vi "AB_RW_Project_Build_Info.vi"(7 "action":T1, 8 "error in (no error)":errorcluster, 10 "buildInfo in":T2, 11 "Object In":T3) -> (0 "error out":errorcluster, 2 "buildInfo out":T2, 3 "Object Out":T3)   [LabVIEW 2020]
uses:
  <resource>/Framework/Providers/API/ItemRef.ctl
  <vilib>/AppBuilder/RW_Project/AB_RW_Project_Build_Data.ctl
  <vilib>/AppBuilder/RW_Project/AB_RW_Project_PropBag_Action.ctl
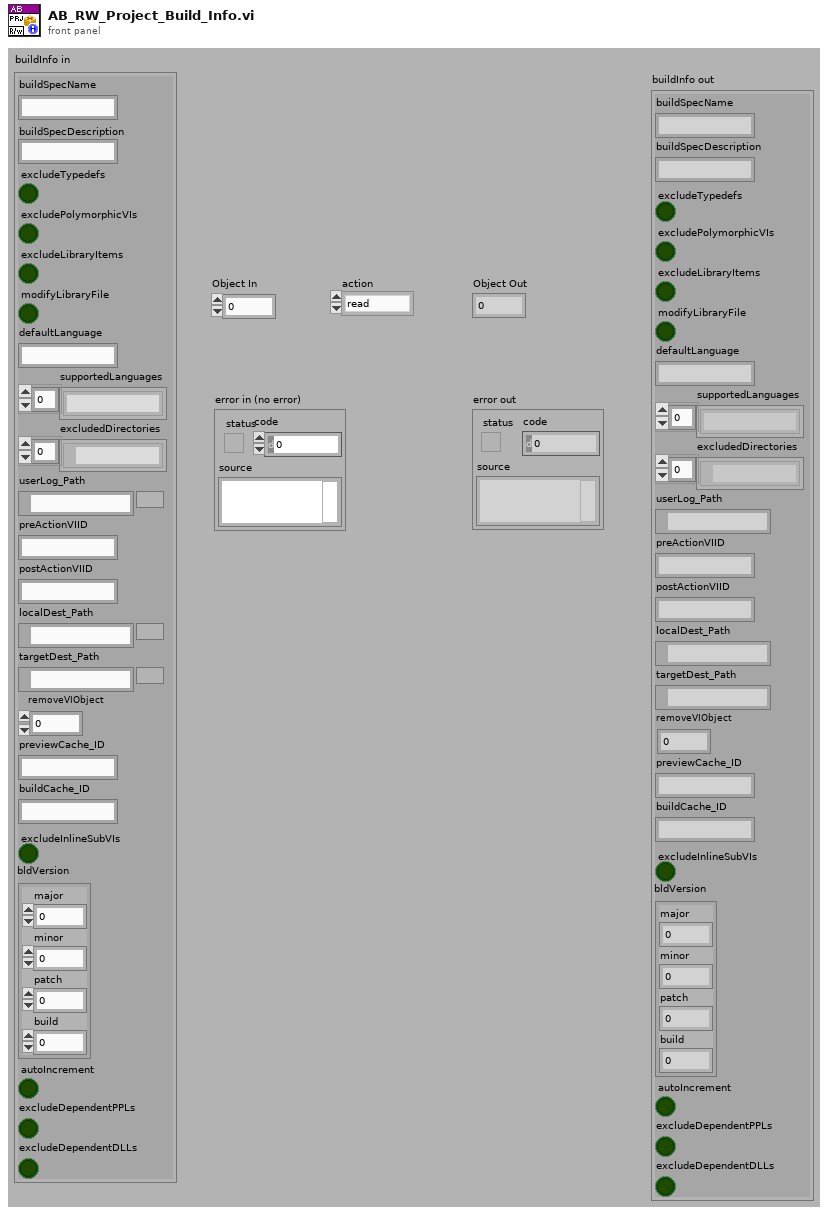
[diagram p1: front panel]
types:
  T1 = typedef "AB_RW_Project_PropBag_Action.ctl" = enum16{"read", "write", "clear", "readPrevious", "writePrevious", "clearPrevious"}
  T2 = typedef "AB_RW_Project_Build_Data.ctl" = cluster{"buildSpecName":string, "buildSpecDescription":string, "excludeTypedefs":bool, "excludePolymorphicVIs":bool, "excludeLibraryItems":bool, "modifyLibraryFile":bool, "defaultLanguage":string, "supportedLanguages":string[], "excludedDirectories":path[], "userLog_Path":path, "preActionVIID":string, "postActionVIID":string, "localDest_Path":path, "targetDest_Path":path, "removeVIObject":u16, "previewCache_ID":string, "buildCache_ID":string, "excludeInlineSubVIs":bool, "bldVersion":cluster{"major":u16, "minor":u16, "patch":u16, "build":u16}, "autoIncrement":bool, "excludeDependentPPLs":bool, "excludeDependentDLLs":bool}
  T3 = typedef "ItemRef.ctl" = u64
  T4 = cluster{"[0]":i32, "[1]":i32, "[2]":i32, "[3]":i32}
  T5 = cluster{"major":u16, "minor":u16, "patch":u16, "build":u16}
  T6 = typedef "AB_Relative_Path_Type.ctl" = enum16{"<none>", "relativeToCommon", "relativeToAppDir", "relativeToProject"}
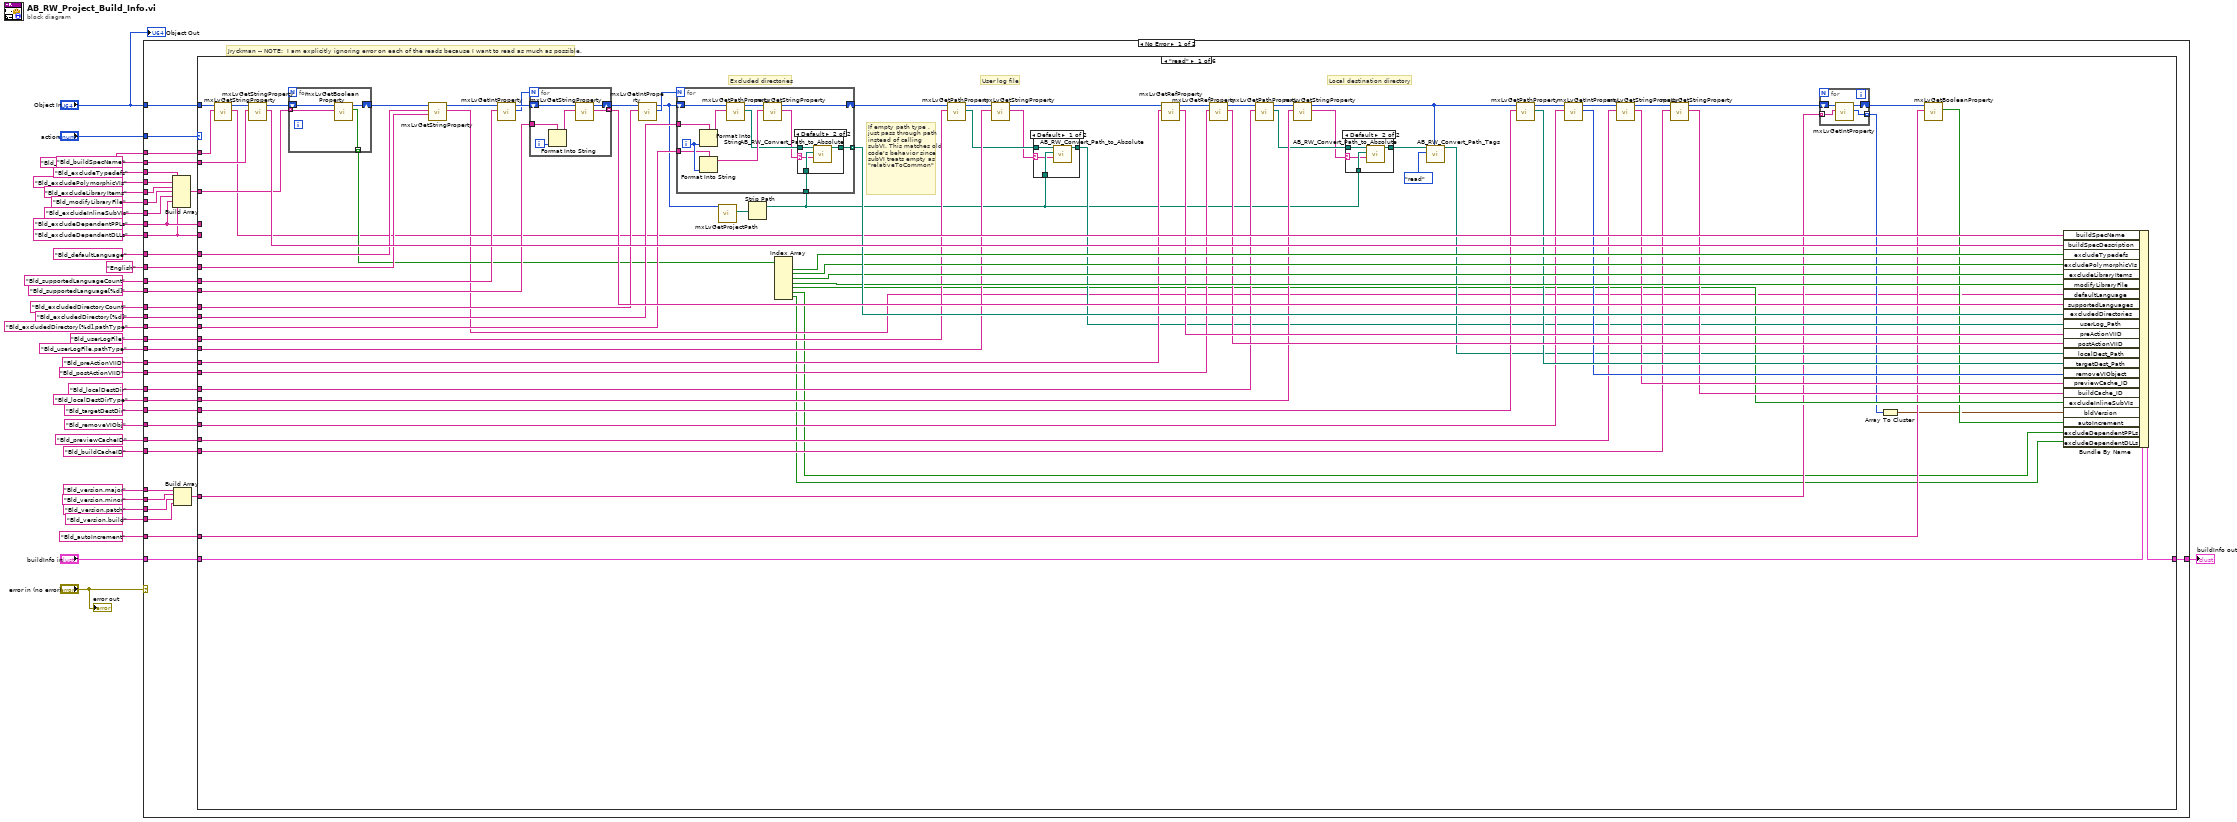
[diagram p0: block diagram]
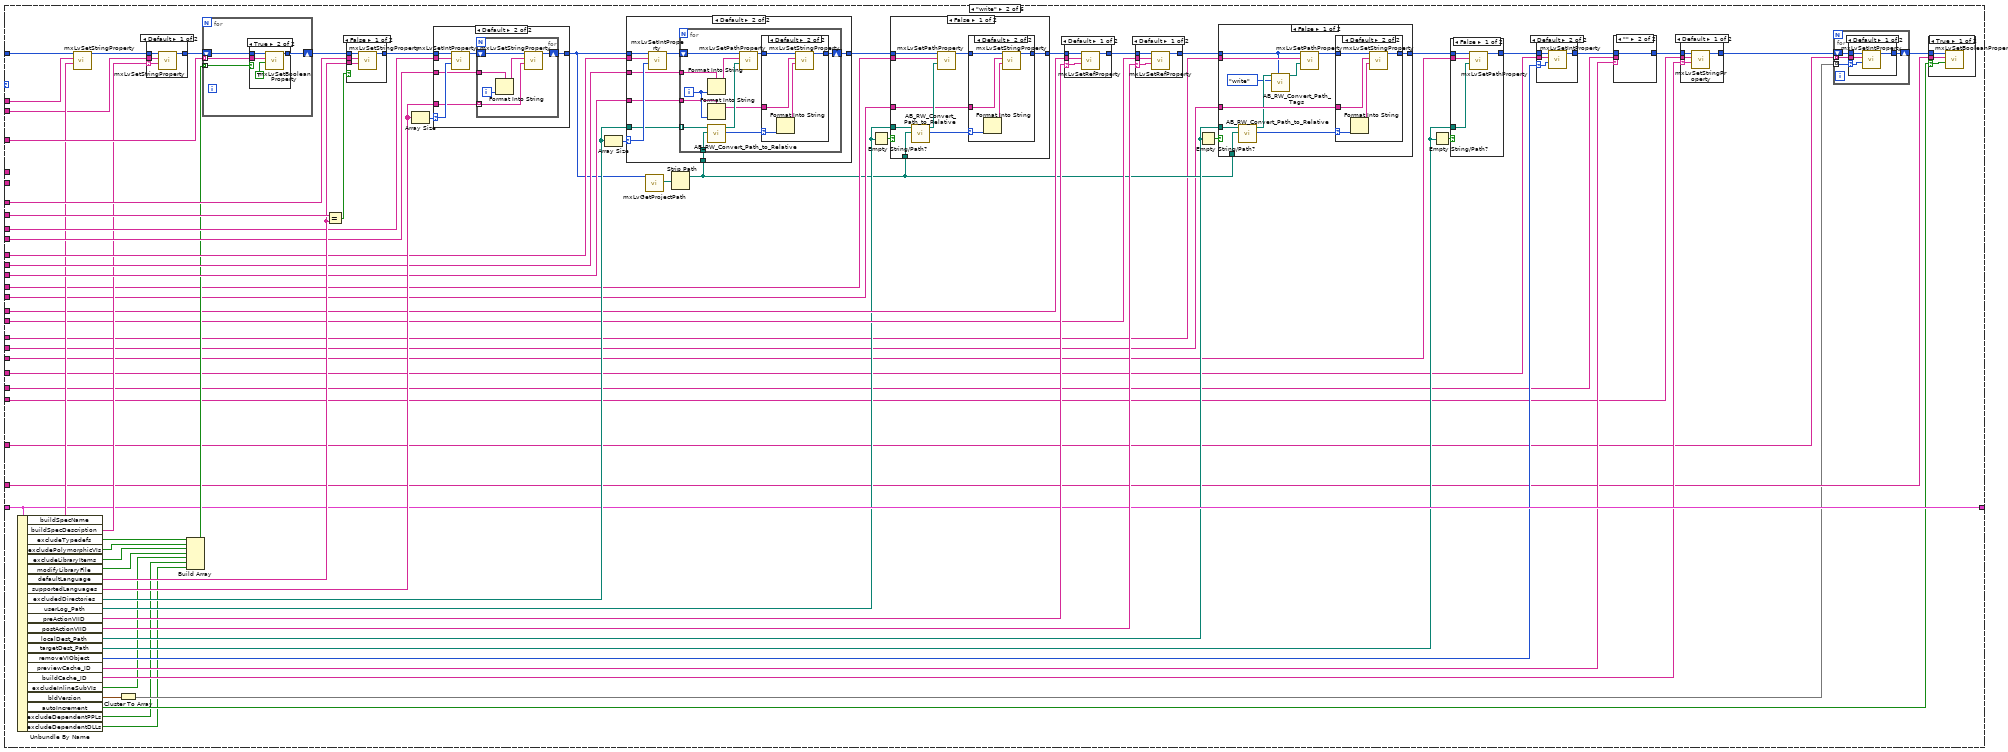
[diagram p5: hidden frame]
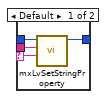
[diagram p9: hidden frame]
diagram:
  n1 = case shown="No Error" "error in (no error)" {
    tunnel: "Object In" -> [w73 _]
    tunnel: [w62 _] -> w34
    tunnel: "Bld_buildSpecDescription" ("Tag") -> [w72 _]
    tunnel: "Bld_excludeTypedefs" ("Tag") -> [w58 _]
    tunnel: "Bld_defaultLanguage" ("Tag") -> [w71 _]
    tunnel: "English" ("Tag") -> [w70 _]
    tunnel: "Bld_supportedLanguageCount" ("Tag") -> [w69 _]
    tunnel: "Bld_supportedLanguage[%d]" ("Tag") -> [w68 _]
    tunnel: "Bld_excludedDirectoryCount" ("Tag") -> [w67 _]
    tunnel: "Bld_excludedDirectory[%d]" ("Tag") -> [w66 _]
    tunnel: "Bld_excludedDirectory[%d].pathType" ("Tag") -> [w65 _]
    tunnel: "buildInfo in" -> [w64 _]
    tunnel: "action" -> [w63 _]
    tunnel: "Bld_excludePolymorphicVIs" ("Tag") -> [w61 _]
    tunnel: "Bld_excludeLibraryItems" ("Tag") -> [w60 _]
    tunnel: "Bld_modifyLibraryFile" ("Tag") -> [w59 _]
    tunnel: "Bld_buildSpecName" ("Tag") -> [w56 _]
    tunnel: "Bld_userLogFile" ("Tag") -> [w55 _]
    tunnel: "Bld_userLogFile.pathType" ("Tag") -> [w54 _]
    tunnel: "Bld_preActionVIID" ("Tag") -> [w53 _]
    tunnel: "Bld_postActionVIID" ("Tag") -> [w52 _]
    tunnel: "Bld_localDestDir" ("Tag") -> [w51 _]
    tunnel: "Bld_targetDestDir" ("Tag") -> [w50 _]
    tunnel: "Bld_localDestDirType" ("Tag") -> [w49 _]
    tunnel: "Bld_removeVIObj" ("Tag") -> [w48 _]
    tunnel: "Bld_previewCacheID" ("Tag") -> [w47 _]
    tunnel: "Bld_buildCacheID" ("Tag") -> [w46 _]
    tunnel: "Bld_excludeInlineSubVIs" ("Tag") -> [w45 _]
    tunnel: "Bld_version.major" ("Tag") -> [w43 _]
    tunnel: "Bld_version.minor" ("Tag") -> [w42 _]
    tunnel: "Bld_version.patch" ("Tag") -> [w40 _]
    tunnel: "Bld_version.build" ("Tag") -> [w41 _]
    tunnel: "Bld_autoIncrement" ("Tag") -> [w44 _]
    tunnel: "Bld_excludeDependentPPLs" ("Tag") -> [w38 _]
    tunnel: "Bld_excludeDependentDLLs" ("Tag") -> [w37 _]
    frame No Error {
      # "Jryckman -- NOTE:  I am explicitly ignoring error on each of the reads because I want to read as much as possible."
      n2 = Build Array(w58, w61, w60, w59, w45, w38, w37) -> (w57:string[])
      n3 = Build Array(w43, w42, w40, w41) -> (w39:string[])
      n4 = case shown="\"read\"" w63 {
        tunnel: w73 -> [w125 w242 w440 w465 w470 w483]
        tunnel: w72 -> [w151 w237 w442 _ _ _]
        tunnel: w71 -> [w149 w262 w441 _ _ _]
        tunnel: w70 -> [w148 w261 _ _ _ _]
        tunnel: w69 -> [w146 w256 w439 _ _ _]
        tunnel: w68 -> [w143 w255 w436 _ _ _]
        tunnel: w67 -> [w140 w251 w432 _ _ _]
        tunnel: w66 -> [w138 w250 w431 _ _ _]
        tunnel: w65 -> [w137 w249 w430 _ _ _]
        tunnel: w64 -> [w134 w221 w427 w467 w471 w484]
        tunnel: [w135 w221 w427 w466 w471 w484] -> w62
        tunnel: w57 -> [w131 w243 w426 _ _ _]
        tunnel: w56 -> [w123 w240 w425 _ _ _]
        tunnel: w55 -> [w118 w234 w423 _ _ _]
        tunnel: w54 -> [w116 w230 w421 _ _ _]
        tunnel: w53 -> [w115 w228 w418 _ _ _]
        tunnel: w52 -> [w112 w225 w417 _ _ _]
        tunnel: w51 -> [w107 w216 w414 _ _ _]
        tunnel: w50 -> [w105 w214 w412 _ _ _]
        tunnel: w49 -> [w106 w217 w413 _ _ _]
        tunnel: w48 -> [w101 w210 w409 w464 w469 w482]
        tunnel: w47 -> [w99 w207 w407 _ _ _]
        tunnel: w46 -> [w96 w204 w405 _ _ _]
        tunnel: w44 -> [w79 w198 w401 _ _ _]
        tunnel: w39 -> [w81 w195 w403 _ _ _]
        tunnel: w38 -> [_ _ _ _ _ w479]
        tunnel: w37 -> [_ _ _ _ _ w478]
        frame "read" {
          # "If empty path type , just pass through path instead of calling subVI. This matches old code's behavior since subVI treats empty as \"relativeToCommon\""
          # "Local destination directory"
          # "User log file"
          # "Excluded directories"
          n5 = call <resource>:"mxLvGetStringProperty.vi"("Tag"=w123, "Item"=w125) -> ("Value"=w122:string, "Item"=w124:T3)  [unwired: 1 in, 7 out]
          n6 = call <resource>:"mxLvGetStringProperty.vi"("Tag"=w151, "Item"=w124) -> ("Value"=w150:string, "Item"=w133:T3)  [unwired: 1 in, 7 out]
          n7 = for {
            shift-right: [w169] -> w132
            shift-left: w133 -> [w167]
            tunnel: w131 -> [w168] mode=indexing
            tunnel: [w166] -> w130 mode=indexing
            n8 = call <resource>:"mxLvGetBooleanProperty.vi"("Tag"=w168, "Item"=w167) -> ("Value"=w166:bool, "Item"=w169:T3)  [unwired: 1 in, 7 out]
          }
          n9 = call <resource>:"mxLvGetStringProperty.vi"("Default Value (\"\")"=w148, "Tag"=w149, "Item"=w132) -> ("Value"=w76:string, "Item"=w147:T3)  [unwired: 1 in, 6 out]
          n10 = call <resource>:"mxLvGetIntProperty.vi"("Tag"=w146, "Item"=w147) -> ("Value"=w144:i32, "Item"=w145:T3)  [unwired: 1 in, 7 out]
          n11 = for {
            N: w144 -> [_]
            shift-right: [w189] -> w141
            shift-left: w145 -> [w190]
            tunnel: w143 -> [w191]
            tunnel: [w187] -> w142 mode=indexing
            i -> [w192]
            n12 = Format Into String(format string=w191, w192) -> (resulting string=w188:string)  [unwired: 2 in, 1 out]
            n13 = call <resource>:"mxLvGetStringProperty.vi"("Tag"=w188, "Item"=w190) -> ("Value"=w187:string, "Item"=w189:T3)  [unwired: 1 in, 7 out]
          }
          n14 = call <resource>:"mxLvGetIntProperty.vi"("Tag"=w140, "Item"=w141) -> ("Value"=w139:i32, "Item"=w121:T3)  [unwired: 1 in, 7 out]
          n15 = call <resource>:"mxLvGetProjectPath.vi"("Item"=w121) -> ("Project Path"=w120:path)  [unwired: 1 in, 9 out]
          n16 = Strip Path(path=w120) -> (stripped path=w86:path)  [unwired: 1 out]
          n17 = for {
            N: w139 -> [_]
            shift-right: [w174] -> w119
            shift-left: w121 -> [w178]
            tunnel: w138 -> [w181]
            tunnel: w137 -> [w179]
            tunnel: w86 -> [w171]
            tunnel: [w172] -> w136 mode=indexing
            i -> [w180]
            n18 = Format Into String(format string=w181, w180) -> (resulting string=w177:string)  [unwired: 2 in, 1 out]
            n19 = Format Into String(format string=w179, w180) -> (resulting string=w175:string)  [unwired: 2 in, 1 out]
            n20 = call <resource>:"mxLvGetPathProperty.vi"("Tag"=w177, "Item"=w178) -> ("Path"=w173:path, "Item"=w176:T3)  [unwired: 2 in, 6 out]
            n21 = call <resource>:"mxLvGetStringProperty.vi"("Tag"=w175, "Item"=w176) -> ("Value"=w170:string, "Item"=w174:T3)  [unwired: 1 in, 7 out]
            n22 = case shown="Default" w170 {
              selector: w170 -> [_ w183]
              tunnel: w173 -> [w182 w186]
              tunnel: [w182 w185] -> w172
              tunnel: w171 -> [_ w184]
              frame "" {
              }
              frame Default {
                n23 = call <vilib>:"AB_RW_Convert_Path_to_Absolute.vi"("relativeType"=w183, "commonPath"=w184, "relativePath"=w186) -> ("absolute path"=w185:path)  [unwired: 7 in, 1 out]
              }
            }
          }
          n24 = Index Array(array=w130) -> (element #1=w129:bool, element #2=w128:bool, element #3=w127:bool, element #4=w126:bool, element #5=w83:bool, element #6=w74:bool, element #7=w75:bool)  [unwired: 7 in]
          n25 = call <resource>:"mxLvGetPathProperty.vi"("Tag"=w118, "Item"=w119) -> ("Path"=w90:path, "Item"=w117:T3)  [unwired: 2 in, 6 out]
          n26 = call <resource>:"mxLvGetStringProperty.vi"("Tag"=w116, "Item"=w117) -> ("Value"=w85:string, "Item"=w114:T3)  [unwired: 1 in, 7 out]
          n27 = case shown="Default" w85 {
            selector: w85 -> [w161 _]
            tunnel: w90 -> [w164 w165]
            tunnel: [w163 w165] -> w89
            tunnel: w86 -> [w162 _]
            frame Default {
              n28 = call <vilib>:"AB_RW_Convert_Path_to_Absolute.vi"("relativeType"=w161, "commonPath"=w162, "relativePath"=w164) -> ("absolute path"=w163:path)  [unwired: 7 in, 1 out]
            }
            frame "" {
            }
          }
          n29 = call <resource>:"mxLvGetRefProperty.vi"("Tag"=w115, "Item"=w114) -> ("Value"=w113:string, "Item"=w111:T3)  [unwired: 1 in, 7 out]
          n30 = call <resource>:"mxLvGetRefProperty.vi"("Tag"=w112, "Item"=w111) -> ("Value"=w110:string, "Item"=w108:T3)  [unwired: 1 in, 7 out]
          n31 = call <resource>:"mxLvGetPathProperty.vi"("Tag"=w107, "Item"=w108) -> ("Path"=w88:path, "Item"=w109:T3)  [unwired: 2 in, 6 out]
          n32 = call <resource>:"mxLvGetStringProperty.vi"("Tag"=w106, "Item"=w109) -> ("Value"=w84:string, "Item"=w92:T3)  [unwired: 1 in, 7 out]
          n33 = case shown="Default" w84 {
            selector: w84 -> [_ w157]
            tunnel: w88 -> [w156 w160]
            tunnel: [w156 w159] -> w87
            tunnel: w86 -> [_ w158]
            frame "" {
            }
            frame Default {
              n34 = call <vilib>:"AB_RW_Convert_Path_to_Absolute.vi"("relativeType"=w157, "commonPath"=w158, "relativePath"=w160) -> ("absolute path"=w159:path)  [unwired: 7 in, 1 out]
            }
          }
          n35 = call <vilib>:"AB_RW_Convert_Path_Tags.vi"("buildObject"=w92, "action"=AB_RW_Project_PropBag_Action."read", "Path in"=w87) -> ("Path out"=w93:path)  [unwired: 1 in, 7 out]
          n36 = call <resource>:"mxLvGetPathProperty.vi"("Tag"=w105, "Item"=w92) -> ("Path"=w104:path, "Item"=w103:T3)  [unwired: 2 in, 6 out]
          n37 = call <resource>:"mxLvGetIntProperty.vi"("Tag"=w101, "Item"=w103) -> ("Value"=w102:i32, "Item"=w100:T3)  [unwired: 7 in, 1 out]
          n38 = call <resource>:"mxLvGetStringProperty.vi"("Tag"=w99, "Item"=w100) -> ("Value"=w98:string, "Item"=w97:T3)  [unwired: 1 in, 7 out]
          n39 = call <resource>:"mxLvGetStringProperty.vi"("Tag"=w96, "Item"=w97) -> ("Value"=w95:string, "Item"=w94:T3)  [unwired: 1 in, 7 out]
          n40 = for {
            shift-right: [w154] -> w80
            shift-left: w94 -> [w155]
            tunnel: w81 -> [w152] mode=indexing
            tunnel: [w153] -> w82 mode=indexing
            n41 = call <resource>:"mxLvGetIntProperty.vi"("Tag"=w152, "Item"=w155) -> ("Value"=w153:i32, "Item"=w154:T3)  [unwired: 1 in, 7 out]
          }
          n42 = Array To Cluster(array=w82) -> (cluster=w77:T4)
          n43 = call <resource>:"mxLvGetBooleanProperty.vi"("Tag"=w79, "Item"=w80) -> ("Value"=w78:bool)  [unwired: 1 in, 8 out]
          n44 = Bundle By Name(cluster=w134, "buildSpecName"=w122, "buildSpecDescription"=w150, "excludeTypedefs"=w129, "excludePolymorphicVIs"=w128, "excludeLibraryItems"=w127, "modifyLibraryFile"=w126, "defaultLanguage"=w76, "supportedLanguages"=w142, "excludedDirectories"=w136, "userLog_Path"=w89, "preActionVIID"=w113, "postActionVIID"=w110, "localDest_Path"=w93, "targetDest_Path"=w104, "removeVIObject"=w102, "previewCache_ID"=w98, "buildCache_ID"=w95, "excludeInlineSubVIs"=w83, "bldVersion"=w77, "autoIncrement"=w78, "excludeDependentPPLs"=w74, "excludeDependentDLLs"=w75) -> (w135:T2)
        }
        frame "write" {
          n45 = Unbundle By Name(w221) -> ("buildSpecName"=w241:string, "buildSpecDescription"=w236:string, "excludeTypedefs"=w248:bool, "excludePolymorphicVIs"=w247:bool, "excludeLibraryItems"=w246:bool, "modifyLibraryFile"=w245:bool, "defaultLanguage"=w260:string, "supportedLanguages"=w254:string[], "excludedDirectories"=w252:path[], "userLog_Path"=w220:path, "preActionVIID"=w227:string, "postActionVIID"=w224:string, "localDest_Path"=w219:path, "targetDest_Path"=w213:path, "removeVIObject"=w209:u16, "previewCache_ID"=w206:string, "buildCache_ID"=w203:string, "excludeInlineSubVIs"=w201:bool, "bldVersion"=w197:T5, "autoIncrement"=w199:bool, "excludeDependentPPLs"=w194:bool, "excludeDependentDLLs"=w193:bool)
          n46 = call <resource>:"mxLvSetStringProperty.vi"("Value (\"\")"=w241, "Tag"=w240, "Item"=w242) -> ("Item"=w239:T3)  [unwired: 2 in, 6 out]
          n47 = Cluster To Array(cluster=w197) -> (array=w196:u16[])
          n48 = case shown="Default" w236 {
            selector: w236 -> [w340 _]
            tunnel: w239 -> [w343 w344]
            tunnel: w237 -> [w342 _]
            tunnel: [w341 w344] -> w238
            frame Default {
              n49 = call <resource>:"mxLvSetStringProperty.vi"("Value (\"\")"=w340, "Tag"=w342, "Item"=w343) -> ("Item"=w341:T3)  [unwired: 2 in, 6 out]
            }
            frame "" {
            }
          }
          n50 = Build Array(w248, w247, w246, w245, w201, w194, w193) -> (w244:bool[])
          n51 = for {
            shift-right: [w347] -> w263
            shift-left: w238 -> [w348]
            tunnel: w244 -> [w346] mode=indexing
            tunnel: w243 -> [w345] mode=indexing
            n52 = case shown="True" w346 {
              tunnel: w348 -> [w349 w353]
              tunnel: [w349 w352] -> w347
              tunnel: w345 -> [_ w351]
              frame False {
              }
              frame True {
                n53 = call <resource>:"mxLvSetBooleanProperty.vi"("Value (F)"=TRUE, "Tag"=w351, "Item"=w353) -> ("Item"=w352:T3)  [unwired: 2 in, 6 out]
              }
            }
          }
          n54 = Equal?(x=w261, y=w260) -> (x = y?=w259:bool)
          n55 = case shown="False" w259 {
            tunnel: w263 -> [w399 w400]
            tunnel: w262 -> [w398 _]
            tunnel: w260 -> [w397 _]
            tunnel: [w396 w400] -> w257
            frame False {
              n56 = call <resource>:"mxLvSetStringProperty.vi"("Value (\"\")"=w397, "Tag"=w398, "Item"=w399) -> ("Item"=w396:T3)  [unwired: 2 in, 6 out]
            }
            frame True {
            }
          }
          n57 = Array Size(array=w254) -> (size(s)=w258:i32)
          n58 = case shown="Default" w258 {
            selector: w258 -> [_ w387]
            tunnel: w257 -> [w382 w389]
            tunnel: w256 -> [_ w388]
            tunnel: w255 -> [_ w385]
            tunnel: w254 -> [_ w384]
            tunnel: [w382 w383] -> w231
            frame 0 {
            }
            frame Default {
              n59 = call <resource>:"mxLvSetIntProperty.vi"("Value (0)"=w387, "Tag"=w388, "Item"=w389) -> ("Item"=w386:T3)  [unwired: 2 in, 6 out]
              n60 = for {
                shift-right: [w394] -> w383
                shift-left: w386 -> [w395]
                tunnel: w385 -> [w392]
                tunnel: w384 -> [w390] mode=indexing
                i -> [w393]
                n61 = Format Into String(format string=w392, w393) -> (resulting string=w391:string)  [unwired: 2 in, 1 out]
                n62 = call <resource>:"mxLvSetStringProperty.vi"("Value (\"\")"=w390, "Tag"=w391, "Item"=w395) -> ("Item"=w394:T3)  [unwired: 2 in, 6 out]
              }
            }
          }
          n63 = Array Size(array=w252) -> (size(s)=w253:i32)
          n64 = call <resource>:"mxLvGetProjectPath.vi"("Item"=w231) -> ("Project Path"=w232:path)  [unwired: 1 in, 9 out]
          n65 = Strip Path(path=w232) -> (stripped path=w218:path)  [unwired: 1 out]
          n66 = case shown="Default" w253 {
            selector: w253 -> [_ w362]
            tunnel: w231 -> [w354 w357]
            tunnel: w251 -> [_ w363]
            tunnel: w250 -> [_ w360]
            tunnel: w252 -> [_ w359]
            tunnel: w249 -> [_ w358]
            tunnel: [w354 w356] -> w235
            tunnel: w218 -> [_ w355]
            frame 0 {
            }
            frame Default {
              n67 = call <resource>:"mxLvSetIntProperty.vi"("Value (0)"=w362, "Tag"=w363, "Item"=w357) -> ("Item"=w361:T3)  [unwired: 2 in, 6 out]
              n68 = for {
                shift-right: [w375] -> w356
                shift-left: w361 -> [w371]
                tunnel: w360 -> [w374]
                tunnel: w359 -> [w373] mode=indexing
                tunnel: w355 -> [w365]
                tunnel: w358 -> [w364]
                i -> [w369]
                n69 = Format Into String(format string=w374, w369) -> (resulting string=w372:string)  [unwired: 2 in, 1 out]
                n70 = Format Into String(format string=w364, w369) -> (resulting string=w367:string)  [unwired: 2 in, 1 out]
                n71 = call <vilib>:"AB_RW_Convert_Path_to_Relative.vi"("commonPath"=w365, "absolutePath"=w373) -> ("relativeType"=w366:T6, "newPath"=w368:path)  [unwired: 1 in, 7 out]
                n72 = call <resource>:"mxLvSetPathProperty.vi"("Path"=w368, "Tag"=w372, "Item"=w371) -> ("Item"=w370:T3)  [unwired: 2 in, 6 out]
                n73 = case shown="Default" w366 {
                  selector: w366 -> [_ w377]
                  tunnel: [w376 w381] -> w375
                  tunnel: w370 -> [w376 w380]
                  tunnel: w367 -> [_ w378]
                  frame "<none>" {
                  }
                  frame Default {
                    n74 = Format Into String(w377) -> (resulting string=w379:string)  [unwired: 3 in, 1 out]
                    n75 = call <resource>:"mxLvSetStringProperty.vi"("Value (\"\")"=w379, "Tag"=w378, "Item"=w380) -> ("Item"=w381:T3)  [unwired: 2 in, 6 out]
                  }
                }
              }
            }
          }
          n76 = Empty String/Path?(string/path=w220) -> (empty?=w233:bool)
          n77 = case shown="False" w233 {
            tunnel: w235 -> [w332 w339]
            tunnel: w234 -> [w331 _]
            tunnel: w218 -> [w328 _]
            tunnel: w220 -> [w327 _]
            tunnel: w230 -> [w325 _]
            tunnel: [w324 w339] -> w229
            frame False {
              n78 = call <vilib>:"AB_RW_Convert_Path_to_Relative.vi"("commonPath"=w328, "absolutePath"=w327) -> ("relativeType"=w330:T6, "newPath"=w326:path)  [unwired: 1 in, 7 out]
              n79 = call <resource>:"mxLvSetPathProperty.vi"("Path"=w326, "Tag"=w331, "Item"=w332) -> ("Item"=w329:T3)  [unwired: 2 in, 6 out]
              n80 = case shown="Default" w330 {
                selector: w330 -> [_ w335]
                tunnel: w329 -> [w333 w338]
                tunnel: w325 -> [_ w336]
                tunnel: [w333 w334] -> w324
                frame "<none>" {
                }
                frame Default {
                  n81 = Format Into String(w335) -> (resulting string=w337:string)  [unwired: 3 in, 1 out]
                  n82 = call <resource>:"mxLvSetStringProperty.vi"("Value (\"\")"=w337, "Tag"=w336, "Item"=w338) -> ("Item"=w334:T3)  [unwired: 2 in, 6 out]
                }
              }
            }
            frame True {
            }
          }
          n83 = case shown="Default" w227 {
            selector: w227 -> [w320 _]
            tunnel: w229 -> [w322 w323]
            tunnel: w228 -> [w321 _]
            tunnel: [w319 w323] -> w226
            frame Default {
              n84 = call <resource>:"mxLvSetRefProperty.vi"("Value (\"\")"=w320, "Tag"=w321, "Item"=w322) -> ("Item"=w319:T3)  [unwired: 2 in, 6 out]
            }
            frame "" {
            }
          }
          n85 = case shown="Default" w224 {
            selector: w224 -> [w315 _]
            tunnel: w226 -> [w317 w318]
            tunnel: w225 -> [w316 _]
            tunnel: [w314 w318] -> w222
            frame Default {
              n86 = call <resource>:"mxLvSetRefProperty.vi"("Value (\"\")"=w315, "Tag"=w316, "Item"=w317) -> ("Item"=w314:T3)  [unwired: 2 in, 6 out]
            }
            frame "" {
            }
          }
          n87 = Empty String/Path?(string/path=w219) -> (empty?=w223:bool)
          n88 = case shown="False" w223 {
            tunnel: w222 -> [w296 w313]
            tunnel: w216 -> [w306 _]
            tunnel: w218 -> [w303 _]
            tunnel: w219 -> [w302 _]
            tunnel: w217 -> [w301 _]
            tunnel: [w300 w313] -> w215
            frame False {
              n89 = call <vilib>:"AB_RW_Convert_Path_to_Relative.vi"("commonPath"=w303, "absolutePath"=w302) -> ("relativeType"=w305:T6, "newPath"=w299:path)  [unwired: 1 in, 7 out]
              n90 = call <vilib>:"AB_RW_Convert_Path_Tags.vi"("buildObject"=w296, "action"=AB_RW_Project_PropBag_Action."write", "Path in"=w299) -> ("Path out"=w298:path)  [unwired: 1 in, 7 out]
              n91 = call <resource>:"mxLvSetPathProperty.vi"("Path"=w298, "Tag"=w306, "Item"=w296) -> ("Item"=w304:T3)  [unwired: 2 in, 6 out]
              n92 = case shown="Default" w305 {
                selector: w305 -> [_ w309]
                tunnel: w304 -> [w307 w312]
                tunnel: w301 -> [_ w310]
                tunnel: [w307 w308] -> w300
                frame "<none>" {
                }
                frame Default {
                  n93 = Format Into String(w309) -> (resulting string=w311:string)  [unwired: 3 in, 1 out]
                  n94 = call <resource>:"mxLvSetStringProperty.vi"("Value (\"\")"=w311, "Tag"=w310, "Item"=w312) -> ("Item"=w308:T3)  [unwired: 2 in, 6 out]
                }
              }
            }
            frame True {
            }
          }
          n95 = Empty String/Path?(string/path=w213) -> (empty?=w212:bool)
          n96 = case shown="False" w212 {
            tunnel: w215 -> [w294 w295]
            tunnel: w214 -> [w293 _]
            tunnel: w213 -> [w292 _]
            tunnel: [w291 w295] -> w211
            frame False {
              n97 = call <resource>:"mxLvSetPathProperty.vi"("Path"=w292, "Tag"=w293, "Item"=w294) -> ("Item"=w291:T3)  [unwired: 2 in, 6 out]
            }
            frame True {
            }
          }
          n98 = case shown="Default" w209 {
            selector: w209 -> [_ w288]
            tunnel: w211 -> [w286 w290]
            tunnel: w210 -> [_ w287]
            tunnel: [w286 w289] -> w208
            frame 0 {
            }
            frame Default {
              n99 = call <resource>:"mxLvSetIntProperty.vi"("Value (0)"=w288, "Tag"=w287, "Item"=w290) -> ("Item"=w289:T3)  [unwired: 2 in, 6 out]
            }
          }
          n100 = case shown="\"\"" w206 {
            selector: w206 -> [w282 _]
            tunnel: w208 -> [w284 w285]
            tunnel: w207 -> [w283 _]
            tunnel: [w281 w285] -> w205
            frame Default {
              n101 = call <resource>:"mxLvSetStringProperty.vi"("Value (\"\")"=w282, "Tag"=w283, "Item"=w284) -> ("Item"=w281:T3)  [unwired: 2 in, 6 out]
            }
            frame "" {
            }
          }
          n102 = case shown="Default" w203 {
            selector: w203 -> [w277 _]
            tunnel: w205 -> [w279 w280]
            tunnel: w204 -> [w278 _]
            tunnel: [w276 w280] -> w202
            frame Default {
              n103 = call <resource>:"mxLvSetStringProperty.vi"("Value (\"\")"=w277, "Tag"=w278, "Item"=w279) -> ("Item"=w276:T3)  [unwired: 2 in, 6 out]
            }
            frame "" {
            }
          }
          n104 = for {
            tunnel: w196 -> [w269] mode=indexing
            shift-right: [w268] -> w200
            shift-left: w202 -> [w270]
            tunnel: w195 -> [w267] mode=indexing
            n105 = case shown="Default" w269 {
              selector: w269 -> [w273 _]
              tunnel: w270 -> [w274 w275]
              tunnel: w267 -> [w272 _]
              tunnel: [w271 w275] -> w268
              frame Default {
                n106 = call <resource>:"mxLvSetIntProperty.vi"("Value (0)"=w273, "Tag"=w272, "Item"=w274) -> ("Item"=w271:T3)  [unwired: 2 in, 6 out]
              }
              frame 0 {
              }
            }
          }
          n107 = case shown="True" w199 {
            selector: w199 -> [w265 _]
            tunnel: w200 -> [w266 _]
            tunnel: w198 -> [w264 _]
            frame True {
              n108 = call <resource>:"mxLvSetBooleanProperty.vi"("Value (F)"=w265, "Tag"=w264, "Item"=w266) -> ()  [unwired: 2 in, 7 out]
            }
            frame False {
            }
          }
        }
        frame "clear" {
          n109 = Build Array (concatenate)(w425, w442, w426, w441, w439, w432) -> (w428:string[])
          n110 = call <resource>:"mxLvGetIntProperty.vi"("Tag"=w439, "Item"=w440) -> ("Value"=w437:i32, "Item"=w438:T3)  [unwired: 1 in, 7 out]
          n111 = for {
            N: w437 -> [_]
            shift-right: [w458] -> w433
            shift-left: w438 -> [w459]
            tunnel: w436 -> [w460]
            i -> [w461]
            n112 = Format Into String(format string=w460, w461) -> (resulting string=w457:string)  [unwired: 2 in, 1 out]
            n113 = call <resource>:"mxLvDeleteProperty.vi"("Tag"=w457, "Item"=w459) -> ("Item"=w458:T3)  [unwired: 1 in, 8 out]
          }
          n114 = call <resource>:"mxLvGetIntProperty.vi"("Tag"=w432, "Item"=w433) -> ("Value"=w435:i32, "Item"=w434:T3)  [unwired: 1 in, 7 out]
          n115 = for {
            N: w435 -> [_]
            shift-right: [w452] -> w429
            shift-left: w434 -> [w455]
            tunnel: w431 -> [w456]
            tunnel: w430 -> [w450]
            i -> [w451]
            n116 = Format Into String(format string=w456, w451) -> (resulting string=w454:string)  [unwired: 2 in, 1 out]
            n117 = Format Into String(format string=w450, w451) -> (resulting string=w449:string)  [unwired: 2 in, 1 out]
            n118 = call <resource>:"mxLvDeleteProperty.vi"("Tag"=w454, "Item"=w455) -> ("Item"=w453:T3)  [unwired: 1 in, 8 out]
            n119 = call <resource>:"mxLvDeleteProperty.vi"("Tag"=w449, "Item"=w453) -> ("Item"=w452:T3)  [unwired: 1 in, 8 out]
          }
          n120 = for {
            tunnel: w428 -> [w447] mode=indexing
            shift-right: [w446] -> w424
            shift-left: w429 -> [w448]
            n121 = call <resource>:"mxLvDeleteProperty.vi"("Tag"=w447, "Item"=w448) -> ("Item"=w446:T3)  [unwired: 1 in, 8 out]
          }
          n122 = call <resource>:"mxLvDeleteProperty.vi"("Tag"=w423, "Item"=w424) -> ("Item"=w422:T3)  [unwired: 1 in, 8 out]
          n123 = call <resource>:"mxLvDeleteProperty.vi"("Tag"=w421, "Item"=w422) -> ("Item"=w419:T3)  [unwired: 1 in, 8 out]
          n124 = call <resource>:"mxLvDeleteProperty.vi"("Tag"=w418, "Item"=w419) -> ("Item"=w420:T3)  [unwired: 1 in, 8 out]
          n125 = call <resource>:"mxLvDeleteProperty.vi"("Tag"=w417, "Item"=w420) -> ("Item"=w411:T3)  [unwired: 1 in, 8 out]
          n126 = call <resource>:"mxLvDeleteProperty.vi"("Tag"=w414, "Item"=w411) -> ("Item"=w416:T3)  [unwired: 1 in, 8 out]
          n127 = call <resource>:"mxLvDeleteProperty.vi"("Tag"=w413, "Item"=w416) -> ("Item"=w415:T3)  [unwired: 1 in, 8 out]
          n128 = call <resource>:"mxLvDeleteProperty.vi"("Tag"=w412, "Item"=w415) -> ("Item"=w410:T3)  [unwired: 1 in, 8 out]
          n129 = call <resource>:"mxLvDeleteProperty.vi"("Tag"=w409, "Item"=w410) -> ("Item"=w408:T3)  [unwired: 1 in, 8 out]
          n130 = call <resource>:"mxLvDeleteProperty.vi"("Tag"=w407, "Item"=w408) -> ("Item"=w406:T3)  [unwired: 1 in, 8 out]
          n131 = call <resource>:"mxLvDeleteProperty.vi"("Tag"=w405, "Item"=w406) -> ("Item"=w404:T3)  [unwired: 1 in, 8 out]
          n132 = for {
            tunnel: w403 -> [w444] mode=indexing
            shift-right: [w443] -> w402
            shift-left: w404 -> [w445]
            n133 = call <resource>:"mxLvDeleteProperty.vi"("Tag"=w444, "Item"=w445) -> ("Item"=w443:T3)  [unwired: 1 in, 8 out]
          }
          n134 = call <resource>:"mxLvDeleteProperty.vi"("Tag"=w401, "Item"=w402) -> ()  [unwired: 1 in, 9 out]
        }
        frame "readPrevious" {
          # "removeVIObj became an int type due to a new option so convert tag from boolean property to int"
          n135 = call <resource>:"mxLvGetBooleanProperty.vi"("Tag"=w464, "Item"=w465) -> ("Value"=w463:bool)  [unwired: 1 in, 8 out]
          n136 = Boolean To (0,1)(Boolean=w463) -> (0, 1=w462:i16)
          n137 = Bundle By Name(cluster=w467, "removeVIObject"=w462) -> (w466:T2)
        }
        frame "writePrevious" {
          n138 = Unbundle By Name(w471) -> ("removeVIObject"=w468:u16)
          n139 = case shown="1" w468 {
            selector: w468 -> [w473 _]
            tunnel: w470 -> [w475 w477]
            tunnel: w469 -> [w474 w476]
            frame 1 {
              n140 = Greater Than 0?(x=w473) -> (x > 0?=w472:bool)
              n141 = call <resource>:"mxLvSetBooleanProperty.vi"("Value (F)"=w472, "Tag"=w474, "Item"=w475) -> ()  [unwired: 2 in, 7 out]
            }
            frame Default {
              n142 = call <resource>:"mxLvDeleteProperty.vi"("Tag"=w476, "Item"=w477) -> ()  [unwired: 1 in, 9 out]
            }
          }
        }
        frame "clearPrevious" {
          # "Since we are reusing the same property, clear it after reading and before writing it again with the current datatype."
          n143 = call <resource>:"mxLvDeleteProperty.vi"("Tag"=w482, "Item"=w483) -> ("Item"=w481:T3)  [unwired: 1 in, 8 out]
          n144 = call <resource>:"mxLvDeleteProperty.vi"("Tag"=w479, "Item"=w481) -> ("Item"=w480:T3)  [unwired: 1 in, 8 out]
          n145 = call <resource>:"mxLvDeleteProperty.vi"("Tag"=w478, "Item"=w480) -> ()  [unwired: 1 in, 9 out]
        }
      }
    }
    frame Error {
    }
  }
  "buildInfo out" <- w34
  "Object Out" <- "Object In"
  "error out" <- "error in (no error)"
